vi "Get XNET Signal Names.vi"(7 "Parent Ref in":T1 format="%.0x", 8 "error in":errorcluster, 9 "Tree In":refnum<vi>, 10 "Parent":string, 11 "Frms":refnum<k21>[](array[refnum])) -> (0 "error out":errorcluster, 1 "Tree Out":refnum<vi>, 3 "XNET Signal Names":refnum<k21>[](array[refnum]))   [LabVIEW 2019, in "Ghost Bus Addon System Explorer.lvlib"]
uses:
  Ghost Bus Addon System Explorer.lvlib
  <resource>/objmgr/xnet.rc
  <vilib>/NI VeriStand/Custom Device API/Custom Device API.lvlib
  <vilib>/NI VeriStand/Custom Device API/Custom Device Item Ref.ctl
  <vilib>/NI VeriStand/Custom Device API/Custom Device Channel Type.ctl
  <vilib>/NI VeriStand/Custom Device API/Custom Device Channel.ctl
  Addon Shared/SubVIs/GUID Lookup.vi
  Addon Shared/Ghost Bus Addon Shared.lvlib
  <vilib>/NI VeriStand/Custom Device Tools/Custom Device Utility Library/Custom Device Utility Library.lvlib
  <vilib>/NI VeriStand/Custom Device API/Set Item Property (U32).vi
  <vilib>/NI VeriStand/Custom Device Tools/Custom Device Utility Library/NI VeriStand - Search for Item by Name.vi
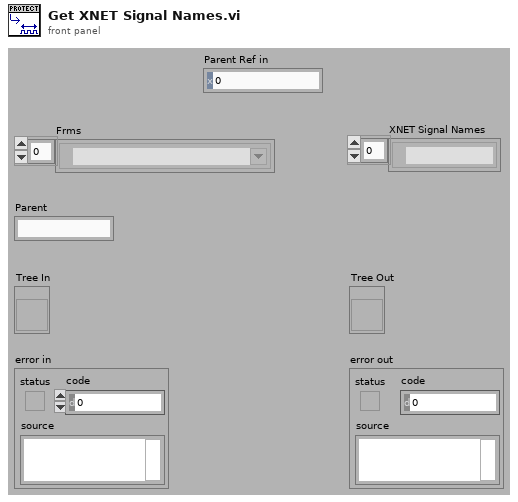
[diagram p1: front panel]
types:
  T1 = typedef "Custom Device API.lvlib/Custom Device Item Ref.ctl" = u64
  T2 = typedef "Custom Device API.lvlib/Custom Device Channel.ctl" = cluster{"Type":T3, "Units":string, "Default Value":dbl, "Faultable":bool, "Scalable":bool}
  T3 = typedef "Custom Device API.lvlib/Custom Device Channel Type.ctl" = enum16{"Input", "Output"}
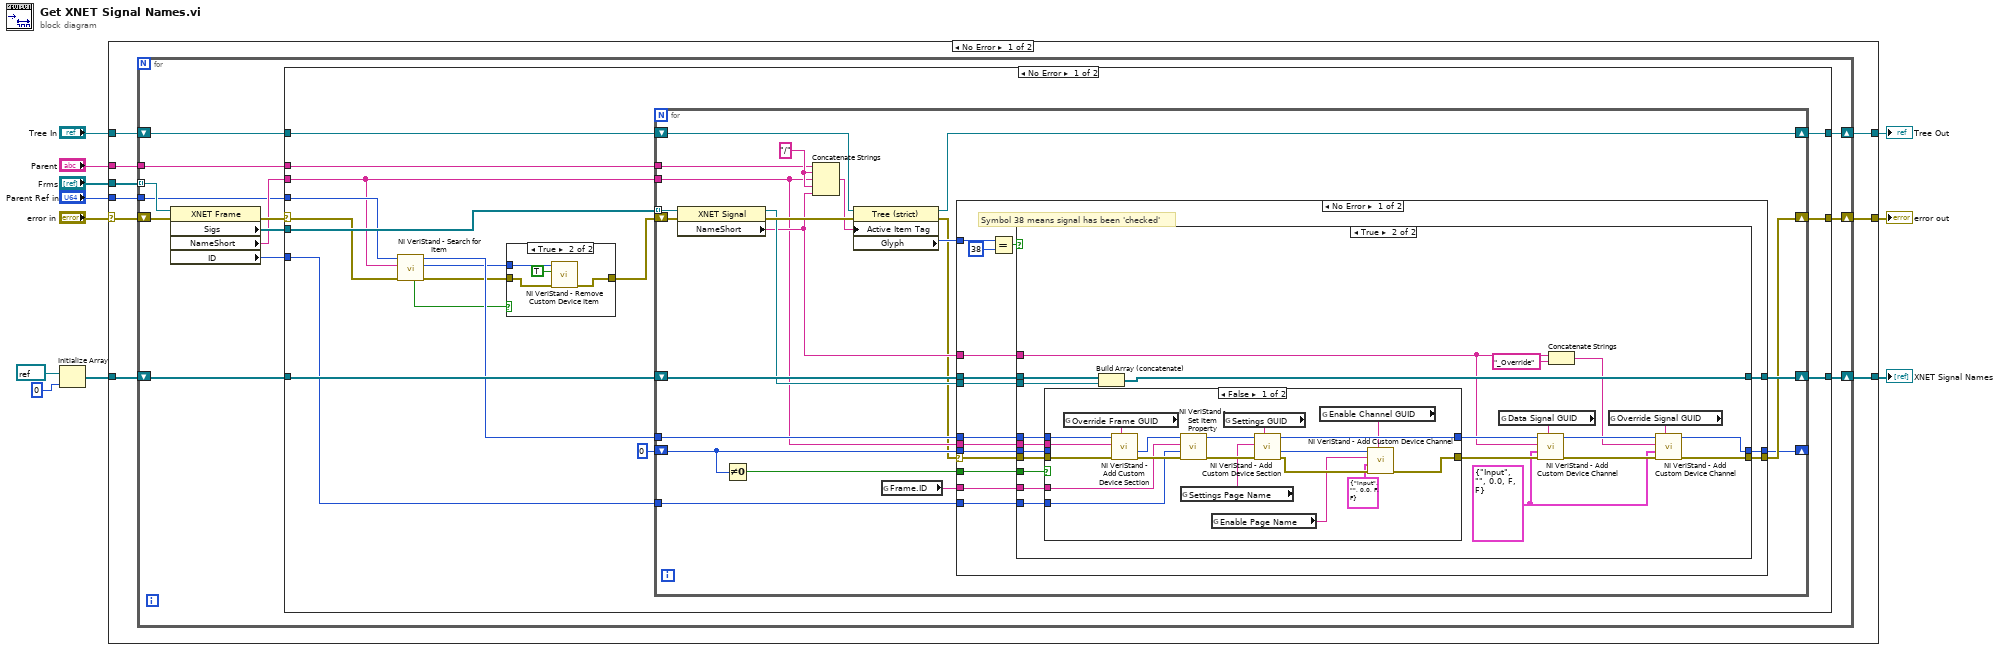
[diagram p0: block diagram]
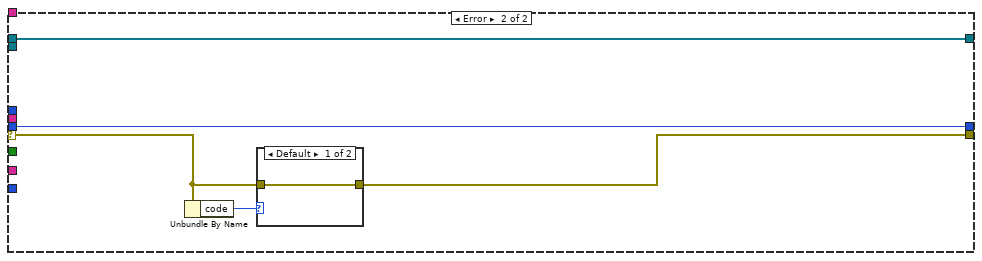
[diagram p5: hidden frame]
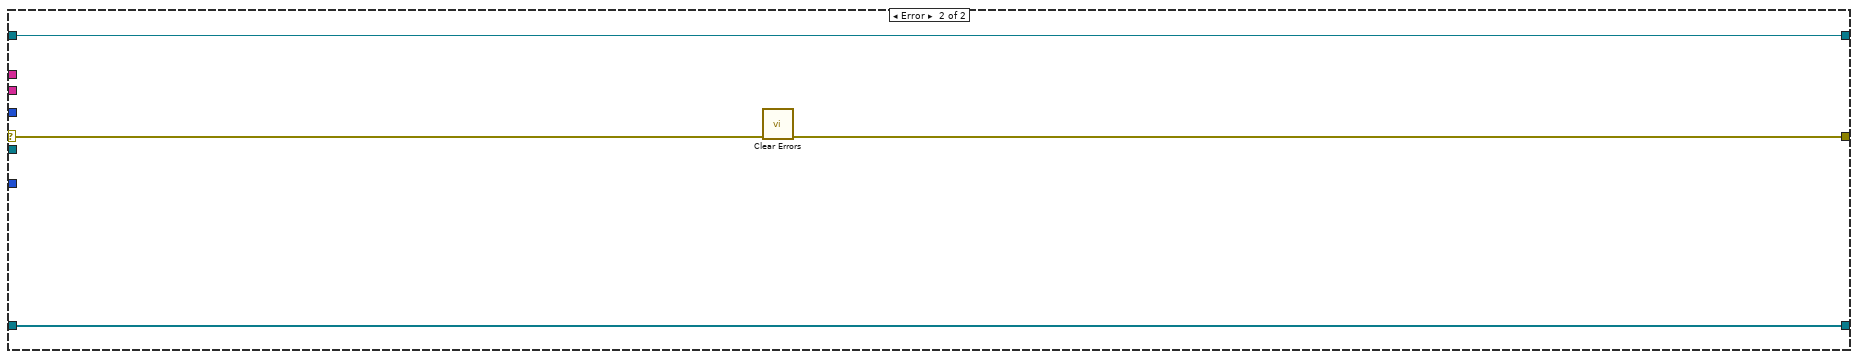
[diagram p7: hidden frame]
diagram:
  n1 = Initialize Array(refnum<k21> refnum ("XNET Signal"), 0 ("dimension size")) -> (w6:refnum<k21>[])
  n2 = case shown="No Error" "error in" {
    selector: "error in" -> [w17 w151]
    tunnel: "Parent" -> [w20 _]
    tunnel: [w19 w151] -> w2
    tunnel: "Frms" -> [w18 _]
    tunnel: [w16 _] -> w8
    tunnel: w6 -> [w15 _]
    tunnel: "Tree In" -> [w14 w150]
    tunnel: [w13 w150] -> w4
    tunnel: "Parent Ref in" -> [w12 _]
    frame No Error {
      n3 = for {
        shift-right: [w30] -> w19
        shift-left: w17 -> [w22]
        tunnel: w18 -> [w33] mode=indexing
        tunnel: w20 -> [w31]
        shift-right: [w27] -> w16
        shift-left: w15 -> [w28]
        shift-right: [w26] -> w13
        shift-left: w14 -> [w29]
        tunnel: w12 -> [w21]
        n4 = property class="XNET Frame"(reference=w33, error in=w22) -> (error out=w25:errorcluster, "Sigs"=w32:refnum<k21>[], "NameShort"=w24:string, "ID"=w23:u32)  [unwired: 1 out]
        n5 = case shown="No Error" w25 {
          selector: w25 -> [w44 w146]
          tunnel: w32 -> [w50 _]
          tunnel: w24 -> [w36 _]
          tunnel: w31 -> [w37 _]
          tunnel: [w34 w147] -> w30
          tunnel: w29 -> [w49 w148]
          tunnel: w28 -> [w48 w149]
          tunnel: [w47 w149] -> w27
          tunnel: [w35 w148] -> w26
          tunnel: w21 -> [w42 _]
          tunnel: w23 -> [w45 _]
          frame No Error {
            n6 = call-poly <vilib>:"NI VeriStand - Search for Item.vi"("error in"=w44, "Item Name"=w36, "Section Ref in"=w42) -> ("error out"=w39:errorcluster, "Item Ref"=w40:T1, "Section Ref out"=w43:T1, "Found"=w41:bool)  [unwired: 5 in]
            n7 = case shown="True" w41 {
              tunnel: w40 -> [_ w55]
              tunnel: w39 -> [w51 w54]
              tunnel: [w51 w53] -> w38
              frame False {
              }
              frame True {
                n8 = call <vilib>:"NI VeriStand - Remove Custom Device Item.vi"("error in (no error)"=w54, "Force Delete (F)"=TRUE, "Item Ref in"=w55) -> ("error out"=w53:errorcluster)  [unwired: 7 in, 1 out]
              }
            }
            n9 = for {
              tunnel: w50 -> [w77] mode=indexing
              tunnel: w36 -> [w59]
              tunnel: w37 -> [w74]
              shift-right: [w66] -> w34
              shift-left: w38 -> [w76]
              shift-right: [w70] -> w47
              shift-left: w48 -> [w69]
              shift-right: [w67] -> w35
              shift-left: w49 -> [w72]
              tunnel: w43 -> [w65]
              shift-right: [w64] -> _
              shift-left: T1 0 ("Parent Ref out") -> [w63]
              tunnel: w45 -> [w60]
              w75 = "/" ("string")
              n10 = property class="XNET Signal"(reference=w77, error in=w76) -> (reference out=w68:refnum<k21>, error out=w73:errorcluster, "NameShort"=w61:string)
              n11 = Not Equal To 0?(x=w63) -> (x != 0?=w62:bool)
              n12 = Concatenate Strings(w74, w75, w59, w75, w61) -> (w56:string)
              n13 = property class="Tree (strict)"(reference=w72, error in=w73, "Active Item Tag"=w56) -> (reference out=w67:refnum<vi>, error out=w58:errorcluster, "Glyph"=w71:i32)
              n14 = global read "GUID Lookup.vi" "Frame.ID"() -> (w57:string)
              n15 = case shown="No Error" w58 {
                selector: w58 -> [w78 w141]
                tunnel: w71 -> [w93 _]
                tunnel: [w90 w143] -> w70
                tunnel: w69 -> [w89 w143]
                tunnel: w68 -> [w88 _]
                tunnel: [w87 w140] -> w66
                tunnel: w65 -> [w86 _]
                tunnel: [w85 w144] -> w64
                tunnel: w63 -> [w84 w144]
                tunnel: w62 -> [w83 _]
                tunnel: w61 -> [w82 _]
                tunnel: w60 -> [w81 _]
                tunnel: w57 -> [w80 _]
                tunnel: w59 -> [w79 _]
                frame No Error {
                  # "Symbol 38 means signal has been 'checked'"
                  n16 = Equal?(x=w93, y=38) -> (x = y?=w91:bool)
                  n17 = case shown="True" w91 {
                    tunnel: [w96 w116] -> w90
                    tunnel: w89 -> [w96 w118]
                    tunnel: w88 -> [_ w117]
                    tunnel: w83 -> [_ w115]
                    tunnel: w79 -> [_ w114]
                    tunnel: w78 -> [w95 w113]
                    tunnel: [w95 w105] -> w87
                    tunnel: w86 -> [_ w112]
                    tunnel: [w94 w103] -> w85
                    tunnel: w84 -> [w94 w111]
                    tunnel: w82 -> [_ w99]
                    tunnel: w81 -> [_ w108]
                    tunnel: w80 -> [_ w107]
                    frame False {
                    }
                    frame True {
                      w100 = T2 {"Type"=enum."Input", "Units"="", "Default Value"=0.0, "Faultable"=FALSE, "Scalable"=FALSE} ("Channel")
                      n18 = case shown="False" w115 {
                        tunnel: w114 -> [w137 _]
                        tunnel: w113 -> [w136 w139]
                        tunnel: [w123 w139] -> w110
                        tunnel: w112 -> [w135 _]
                        tunnel: [w126 w138] -> w109
                        tunnel: w111 -> [_ w138]
                        tunnel: w108 -> [w131 _]
                        tunnel: w107 -> [w132 _]
                        frame False {
                          n19 = global read "GUID Lookup.vi" "Override Frame GUID"() -> (w130:string)
                          n20 = call <vilib>:"NI VeriStand - Add Custom Device Section.vi"("GUID (Default Section)"=w130, "error in (no error)"=w136, "Section Name"=w137, "Parent Ref in"=w135) -> ("error out"=w133:errorcluster, "Section Ptr"=w134:T1)  [unwired: 4 in, 2 out]
                          n21 = call-poly <vilib>:"NI VeriStand - Set Item Property.vi"("error in (no error)"=w133, "Value"=w131, "Property Name"=w132, "Item Ref in"=w134) -> ("error out"=w128:errorcluster, "Item Ref out"=w127:T1)  [unwired: 5 in, 1 out]
                          n22 = global read "GUID Lookup.vi" "Settings Page Name"() -> (w121:string)
                          n23 = global read "GUID Lookup.vi" "Enable Page Name"() -> (w120:string)
                          n24 = global read "GUID Lookup.vi" "Settings GUID"() -> (w129:string)
                          n25 = call <vilib>:"NI VeriStand - Add Custom Device Section.vi"("GUID (Default Section)"=w129, "error in (no error)"=w128, "Section Name"=w121, "Parent Ref in"=w127) -> ("error out"=w124:errorcluster, "Section Ptr"=w125:T1, "Parent Ref out"=w126:T1)  [unwired: 4 in, 1 out]
                          n26 = global read "GUID Lookup.vi" "Enable Channel GUID"() -> (w119:string)
                          n27 = call <vilib>:"NI VeriStand - Add Custom Device Channel.vi"("GUID (Default Channel)"=w119, "error in (no error)"=w124, "Channel"=T2 {"Type"=enum."Input", "Units"="", "Default Value"=0.0, "Faultable"=FALSE, "Scalable"=FALSE}, "Channel Name"=w120, "Parent Ref in"=w125) -> ("error out"=w123:errorcluster)  [unwired: 3 in, 3 out]
                        }
                        frame True {
                        }
                      }
                      n28 = Build Array (concatenate)(w118, w117) -> (w116:refnum<k21>[])
                      n29 = global read "GUID Lookup.vi" "Data Signal GUID"() -> (w102:string)
                      n30 = call <vilib>:"NI VeriStand - Add Custom Device Channel.vi"("GUID (Default Channel)"=w102, "error in (no error)"=w110, "Channel"=w100, "Channel Name"=w99, "Parent Ref in"=w109) -> ("error out"=w106:errorcluster, "Parent Ref out"=w104:T1)  [unwired: 3 in, 2 out]
                      n31 = Concatenate Strings(w99, "_Override" ("string")) -> (w97:string)
                      n32 = global read "GUID Lookup.vi" "Override Signal GUID"() -> (w101:string)
                      n33 = call <vilib>:"NI VeriStand - Add Custom Device Channel.vi"("GUID (Default Channel)"=w101, "error in (no error)"=w106, "Channel"=w100, "Channel Name"=w97, "Parent Ref in"=w104) -> ("error out"=w105:errorcluster, "Parent Ref out"=w103:T1)  [unwired: 3 in, 2 out]
                    }
                  }
                }
                frame Error {
                  n34 = Unbundle By Name(w141) -> ("code"=w142:i32)
                  n35 = case shown="Default" w142 {
                    tunnel: [w145 _] -> w140
                    tunnel: w141 -> [w145 _]
                    frame Default {
                    }
                    frame 1136 {
                    }
                  }
                }
              }
            }
          }
          frame Error {
            n36 = call <vilib>:"Clear Errors.vi"("error in (no error)"=w146) -> ("error out"=w147:errorcluster)  [unwired: 5 in, 1 out]
          }
        }
      }
    }
    frame Error {
    }
  }
  "error out" <- w2
  "XNET Signal Names" <- w8
  "Tree Out" <- w4
